vi "register indicator callbacks.vi"(8 "error in":errorcluster, 9 "controls":refnum<vi>[](array[refnum]), 10 "value index":i32, 11 "displayable in":refnum<class "displayable.lvclass">) -> (0 "error out":errorcluster, 3 "displayable out":refnum<class "displayable.lvclass">)   [LabVIEW 2013, in "displayable.lvclass"]
uses:
  displayable.lvclass
  displayable.lvclass/displayable.ctl
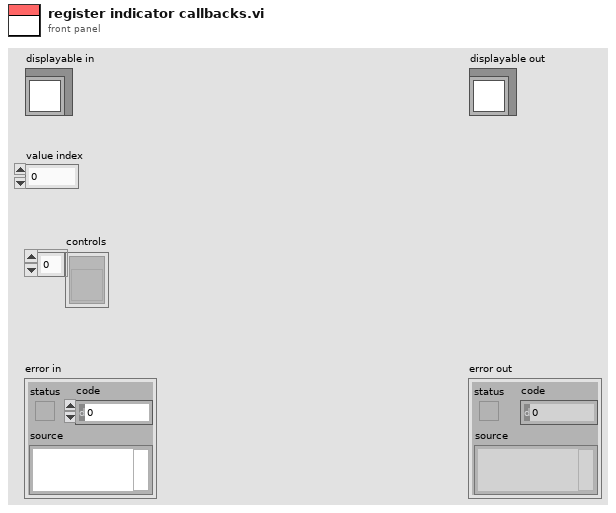
[diagram p1: front panel]
types:
  T1 = typedef "displayable.lvclass/subscription.ctl" = cluster{"control indexes":i32[]}
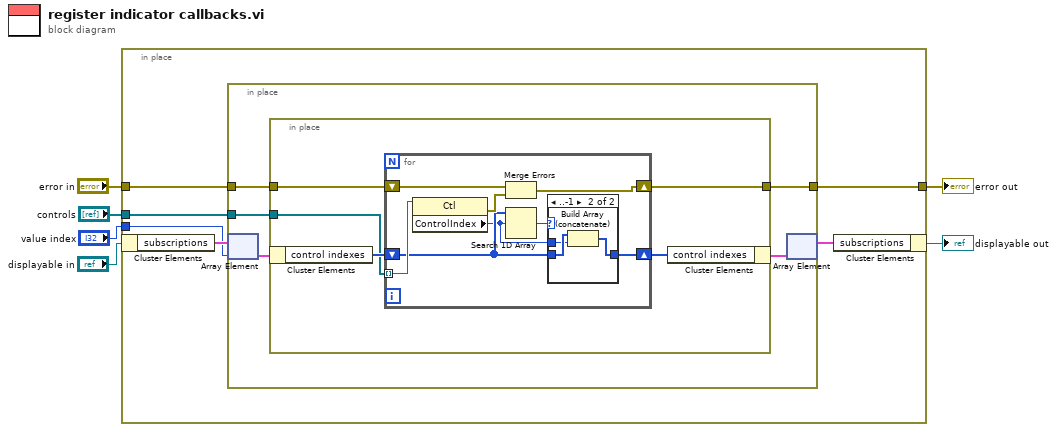
[diagram p0: block diagram]
diagram:
  n1 = in-place {
    in-place-border: "value index" -> [w11]
    in-place-border: [w9] -> w3
    in-place-border: "error in" -> [w8]
    in-place-border: "controls" -> [w7]
    n2 = in-place-cluster #1("displayable in") -> ("subscriptions"=w12:T1[])
    n3 = in-place {
      in-place-border: [w17] -> w9
      in-place-border: w8 -> [w16]
      in-place-border: w7 -> [w13]
      n4 = in-place-array #2(w12, w11) -> (w15:T1)
      n5 = in-place {
        in-place-border: [w18] -> w17
        in-place-border: w16 -> [w19]
        in-place-border: w13 -> [w20]
        n6 = in-place-cluster #3(w15) -> ("control indexes"=w22:i32[])
        n7 = for {
          shift-right: [w24] -> w21
          shift-left: w22 -> [w25]
          tunnel: w20 -> [w30] mode=indexing
          shift-right: [w28] -> w18
          shift-left: w19 -> [w29]
          n8 = property class="Ctl"(reference=w30) -> (error out=w27:errorcluster, "ControlIndex"=w23:i32)  [unwired: 1 in, 1 out]
          n9 = Merge Errors(w29, w27) -> (w28:errorcluster)
          n10 = Search 1D Array(1D array=w25, element=w23) -> (index of element=w26:i32)  [unwired: 1 in]
          n11 = case shown="..-1" w26 {
            tunnel: w25 -> [w31 w34]
            tunnel: [w31 w33] -> w24
            tunnel: w23 -> [_ w32]
            frame 0.. {
            }
            frame ..-1 {
              n12 = Build Array (concatenate)(w34, w32) -> (w33:i32[])
            }
          }
        }
        n13 = in-place-cluster #3("control indexes"=w21) -> (w14:T1)
      }
      n14 = in-place-array #2(w14) -> (w10:T1[])  [unwired: 1 out]
    }
    n15 = in-place-cluster #1("subscriptions"=w10) -> (→"displayable out":refnum<class "displayable.lvclass">)
  }
  "error out" <- w3
